vi "LoadHeaderKenandHerty.vi"(3 "appended path":path, 5 "reference":refnum<vi>) -> (1 "unsuccesful?":bool=TRUE)   [LabVIEW 2009]
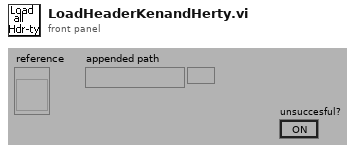
[diagram p1: front panel]
types:
  T1 = enum16{"Display", "change", "Get", "Set", "Set Ken"}
  T2 = typedef "ImageSettings.ctt" = cluster{"Start Position (µm)":cluster{"x":dbl, "y":dbl, "z":dbl}, "End Position (µm)":cluster{"x":dbl, "y":dbl, "z":dbl}, "Image Resolution (nm/pixel)":cluster{"x":dbl, "y":dbl, "z":dbl}, "Image Size (µm)":cluster{"x":dbl, "y":dbl, "z":dbl}, "Image Size (pixel)":cluster{"x":u32, "y":u32, "z":u32}, "Time Resolution\n(ms/pixel)":dbl, "1st Axis":u16, "2nd Axis":u16, "Retrace":bool, "Estimated Time":string}
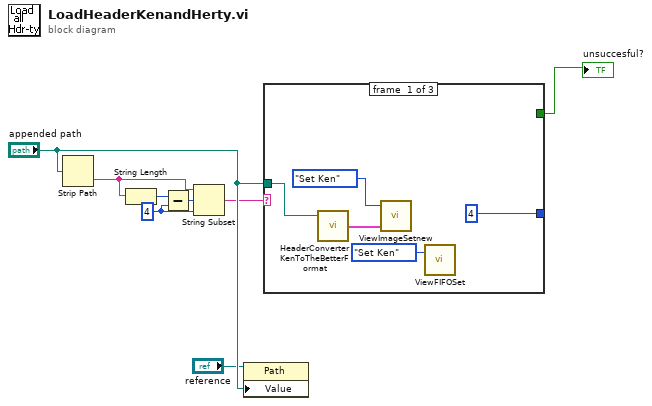
[diagram p0: block diagram]
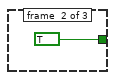
[diagram p2: hidden frame]
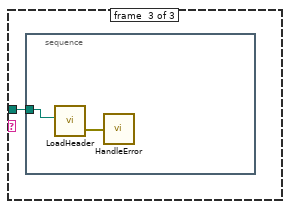
[diagram p3: hidden frame]
diagram:
  w4 = 4 ("y")
  n1 = Strip Path(path="appended path") -> (name=w3:string)  [unwired: 1 out]
  n2 = String Length(string=w3) -> (length=w6:i32)
  n3 = Subtract(x=w6, y=w4) -> (x-y=w5:i32)
  n4 = String Subset(string=w3, offset (0)=w5, length (rest)=w4) -> (substring=w2:string)
  n5 = property on="Property Node" class="Path"(reference="reference", "Value"="appended path") -> ()  [unwired: 1 in, 2 out]
  n6 = case shown="\".hd2\", \".hdr\"" w2 {
    tunnel: "appended path" -> [w11 _ w15]
    tunnel: [4 _ _] -> _
    tunnel: [_ TRUE _] -> w1
    frame #0 {
      n7 = call "HeaderConverterKenToTheBetterFormat.vi"("file path"=w11) -> ("output cluster"=w13:T2)  [unwired: 4 in]
      n8 = call "ViewImageSetnew.vi"("Cluster"=w13, "action"=T1."Set Ken" ("Enum")) -> ()  [unwired: 1 in, 1 out]
      n9 = call "ViewFIFOSet.vi"("Enum"=T1."Set Ken") -> ()  [unwired: 1 in, 1 out]
    }
    frame #1 {
    }
    frame #2 {
      n10 = stacked-sequence {
        tunnel: w15 -> [w16]
        frame #0 {
          n11 = call "LoadHeader.vi"("Path"=w16) -> ("error out"=w17:errorcluster)  [unwired: 4 in]
          n12 = call "HandleError.vi"("error in (no error)"=w17) -> ()
        }
      }
    }
  }
  "unsuccesful?" <- w1
